vi "1111_#PICKUP.vi"(10 "CoPilot":refnum<k33>) -> (3 "CoPilot 2":refnum<k33>)   [LabVIEW 2014]
uses:
  Co-Pilot_game_control.ctl
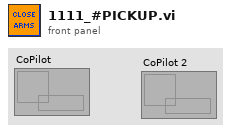
[diagram p1: front panel]
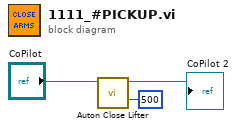
[diagram p0: block diagram]
diagram:
  n1 = call "Auton Close Lifter.vi"("milliseconds to wait"=u32 500, "CoPilot"="CoPilot") -> ("CoPilot 2"=→"CoPilot 2":refnum<k33>)  [unwired: 9 in]
